vi "ReplaceClassReferences.vi"(0 "attribute data":variant, 5 "error in (no error)":errorcluster) -> (14 "attribute data out":variant, 19 "error out":errorcluster)   [LabVIEW 2017, in "G#DebugServer.lvclass"]
doc: "Replaces the class references in the attribute data."
uses:
  <vilib>/addons/_AddQ/G#DebugServer/G#DebugServer.lvclass
  <vilib>/addons/_AddQ/G#Object/G#Object.lvclass
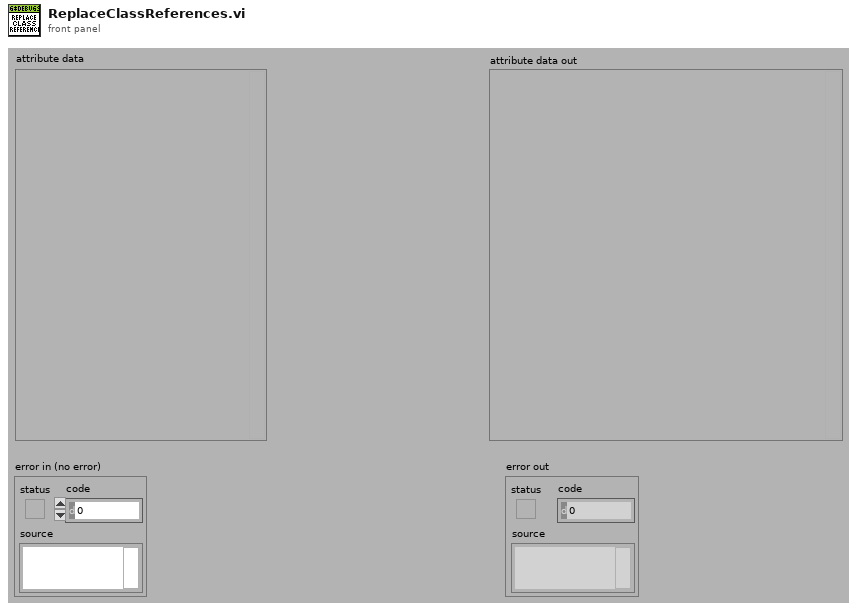
[diagram p1: front panel]
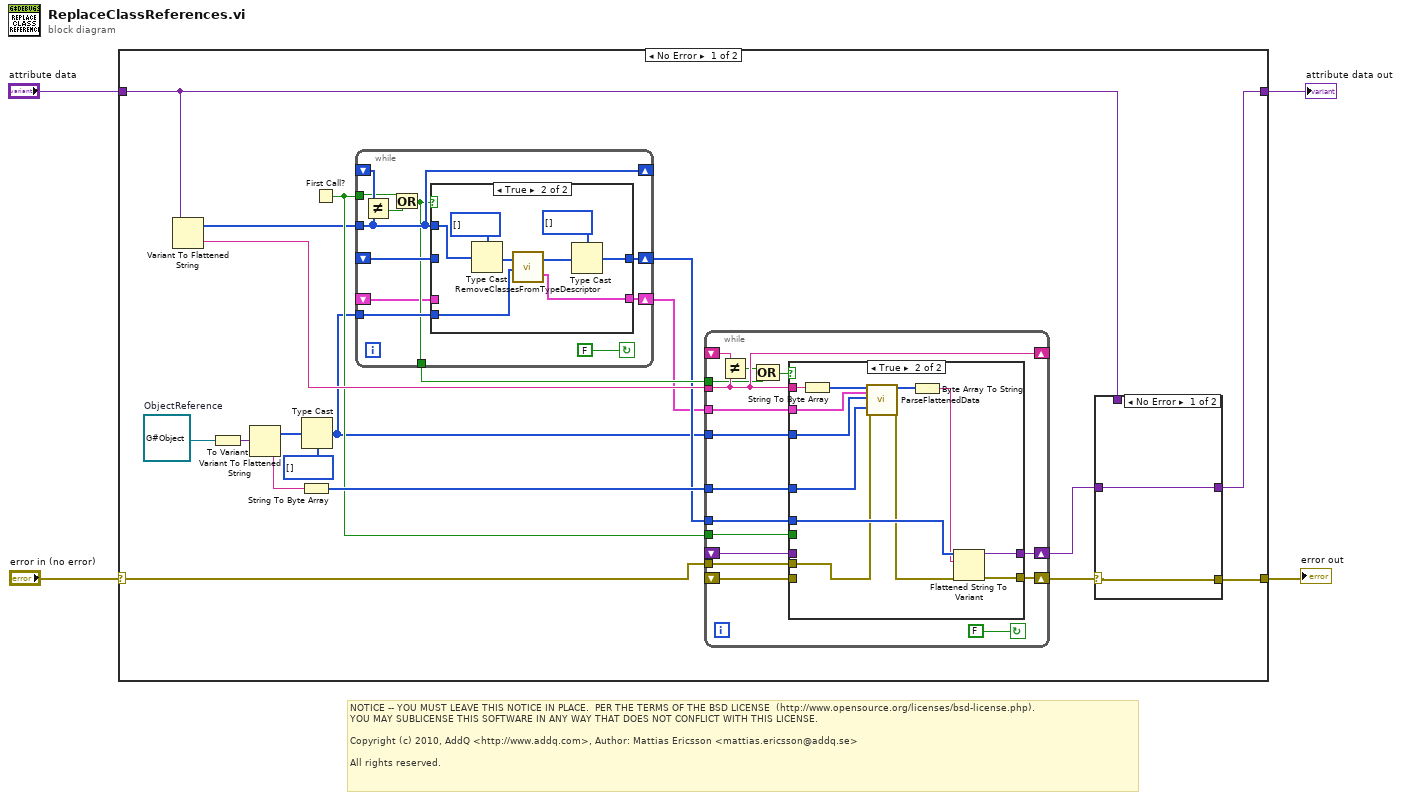
[diagram p0: block diagram]
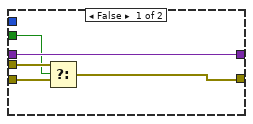
[diagram p2: hidden frame]
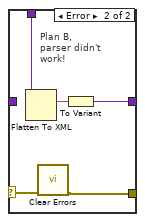
[diagram p3: hidden frame]
diagram:
  # "NOTICE -- YOU MUST LEAVE THIS NOTICE IN PLACE.  PER THE TERMS OF THE BSD LICENSE  (http://www.opensource.org/licenses/bsd-license.php).\nYOU MAY SUBLICENSE THIS SOFTWARE IN ANY WAY THAT DOES NOT CONFLICT WITH THIS LICENSE.\n\nCopyright (c) 2010, AddQ <http://www.addq.com>, Author: Mattias Ericsson <mattias.ericsson@addq.se>\n\nAll rights reserved."
  n1 = case shown="No Error" "error in (no error)" {
    selector: "error in (no error)" -> [w23 w86]
    tunnel: [w22 w86] -> w3
    tunnel: "attribute data" -> [w6 w85]
    tunnel: [w21 w85] -> w1
    frame No Error {
      w5 = refnum<class "G#Object.lvclass"> refnum  # ObjectReference
      n2 = Variant To Flattened String(Variant=w6) -> (data string=w20:string, 1:w8:i16[])
      n3 = To Variant(anything=w5) -> (Variant=w7:variant)
      n4 = Variant To Flattened String(Variant=w7) -> (data string=w12:string, 1:w14:i16[])
      n5 = String To Byte Array(string=w12) -> (unsigned byte array=w19:u8[])
      n6 = Type Cast(type=u8[] [] ("EmptyLabVIEWObjectFlatten"), x=w14) -> (*(type *) &x=w10:u8[])
      n7 = First Call?() -> (First Call?: T/F=w11:bool)
      n8 = while {
        tunnel: w8 -> [w73]
        shift-right: [w73] -> _
        shift-left: _ -> [w74]
        shift-right: [w70] -> w17
        shift-left: _ -> [w69]
        tunnel: w10 -> [w71]
        tunnel: [w68] -> w18
        tunnel: w11 -> [w66]
        shift-right: [w65] -> w9
        shift-left: _ -> [w64]
        stop <- FALSE continue-if-true
        n9 = Not Equal?(x=w74, y=w73) -> (x != y?=w67:bool)
        n10 = Or(x=w66, y=w67) -> (x .or. y?=w68:bool)
        n11 = case shown="True" w68 {
          tunnel: w73 -> [_ w83]
          tunnel: [w76 w79] -> w70
          tunnel: w71 -> [_ w78]
          tunnel: w69 -> [w76 _]
          tunnel: [w75 w77] -> w65
          tunnel: w64 -> [w75 _]
          frame False {
          }
          frame True {
            n12 = Type Cast(type=u8[] [] ("type string"), x=w83) -> (*(type *) &x=w82:u8[])
            n13 = call <vilib>:"RemoveClassesFromTypeDescriptor.vi"("type descriptor"=w82, "replace type desc"=w78) -> ("type descriptor out"=w81:u8[], "type descriptor parsed out"=w77:cluster{"TypeDescr":u8[], "Class":bool}[])  [unwired: 16 in]
            n14 = Type Cast(type=i16[] [] ("type string"), x=w81) -> (*(type *) &x=w79:i16[])
          }
        }
      }
      n15 = while {
        tunnel: w20 -> [w38]
        shift-right: [w38] -> _
        shift-left: _ -> [w39]
        shift-right: [w30] -> w16
        shift-left: _ -> [w37]
        tunnel: w19 -> [w35]
        tunnel: w18 -> [w32]
        tunnel: w17 -> [w31]
        shift-right: [w28] -> w15
        shift-left: _ -> [w29]
        tunnel: w23 -> [w27]
        tunnel: w11 -> [w26]
        tunnel: w9 -> [w25]
        tunnel: w10 -> [w24]
        stop <- FALSE continue-if-true
        n16 = Not Equal?(x=w39, y=w38) -> (x != y?=w33:bool)
        n17 = Compound Arithmetic op=OR(w33, w32) -> (w34:bool)
        n18 = case shown="True" w34 {
          tunnel: w38 -> [_ w51]
          tunnel: w37 -> [w44 _]
          tunnel: w35 -> [_ w55]
          tunnel: w31 -> [_ w54]
          tunnel: [w44 w53] -> w30
          tunnel: w29 -> [w43 _]
          tunnel: [w40 w52] -> w28
          tunnel: w27 -> [w42 w47]
          tunnel: w26 -> [w41 _]
          tunnel: w25 -> [_ w48]
          tunnel: w24 -> [_ w45]
          frame False {
            n19 = Select(t=w42, s=w41, f=w43) -> (s? t:f=w40:errorcluster)
          }
          frame True {
            n20 = String To Byte Array(string=w51) -> (unsigned byte array=w56:u8[])
            n21 = call <vilib>:"ParseFlattenedData.vi"("flattened data"=w56, "type descriptor"=w48, "replace type desc"=w45, "replace object flatten data"=w55, "error in (no error)"=w47) -> ("element data"=w50:u8[], "error out"=w46:errorcluster)  [unwired: 10 in, 3 out]
            n22 = Byte Array To String(unsigned byte array=w50) -> (string=w49:string)
            n23 = Flattened String To Variant(4:w46, 6:w49, 7:w54) -> (0:w52:errorcluster, 3:w53:variant)
          }
        }
      }
      n24 = case shown="No Error" w15 {
        selector: w15 -> [w57 w63]
        tunnel: w16 -> [w58 _]
        tunnel: [w58 w61] -> w21
        tunnel: [w57 w62] -> w22
        tunnel: w6 -> [_ w59]
        frame No Error {
        }
        frame Error {
          # "Plan B,\nparser didn't\nwork!"
          n25 = Flatten To XML(anything=w59) -> (xml string=w60:string)
          n26 = call <vilib>:"Clear Errors.vi"("error in (no error)"=w63) -> ("error out"=w62:errorcluster)  [unwired: 5 in, 1 out]
          n27 = To Variant(anything=w60) -> (Variant=w61:variant)
        }
      }
    }
    frame Error {
    }
  }
  "error out" <- w3
  "attribute data out" <- w1
